vi "altitude.vi"(11 "altitude":dbl[unit]) -> (2 "presure":dbl[unit], 3 "temperature":dbl[unit])   [LabVIEW 2011]
doc: "ÏPOÃPAMMA PAC×ETA ÏAPAMETPOB CTAHÄAPTHOÉ ATMOCÔEPÛ ÃOCT 4401-73"
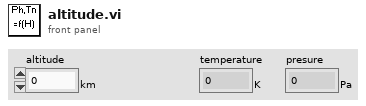
[diagram p1: front panel]
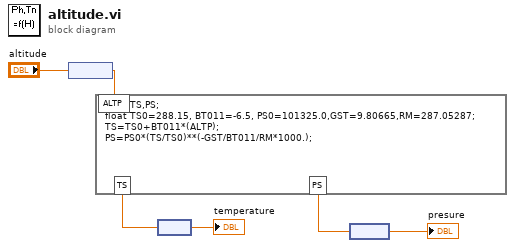
[diagram p0: block diagram]
diagram:
  n1 = node("altitude") -> (w3:dbl)
  n2 = formula code="float TS,PS;\nfloat TS0=288.15, BT011=-6.5, PS0=101325.0,GST=9.80665,RM=287.05287;\nTS=TS0+BT011*(ALTP);                                         \nPS=PS0*(TS/TS0)**(-GST/BT011/RM*1000.);"("ALTP"=w3) -> ("TS"=w5:dbl, "PS"=w4:dbl)
  n3 = node(w5) -> (→"temperature":dbl[unit])
  n4 = node(w4) -> (→"presure":dbl[unit])
